vi "PPAS_Teleop_System_Execute.vi"(11 "Teleop Elapsed Seconds":dbl) -> ()   [LabVIEW 2019]
uses:
  <vilib>/Rock Robotics/WPI/Joystick/XBox Buttons Indexer.ctl
  <vilib>/Rock Robotics/WPI/Joystick/XBox Axes Indexer.ctl
  <vilib>/Rock Robotics/WPI/ThirdParty/JAS_Junk/TrajLib/TypeDef/CHASSIS_SPEEDS.ctl
  <vilib>/Rock Robotics/WPI/ThirdParty/JAS_Junk/TrajLib/VI/Util_GetTime_U32.vi
  <vilib>/Rock Robotics/WPI/ThirdParty/JAS_Junk/TrajLib/VI/numCmd_Send_Generic.vi
  <vilib>/Rock Robotics/WPI/ThirdParty/JAS_Junk/TrajLib/VI/BoolCmd_Send_Internal.vi
  <vilib>/Rock Robotics/WPI/ThirdParty/JAS_Junk/TrajLib/VI/numCmd_ObtainQueue_Generic.vi
  <vilib>/Rock Robotics/WPI/ThirdParty/JAS_Junk/TrajLib/VI/BoolCmd_ObtainQueue.vi
  <vilib>/Rock Robotics/WPI/ThirdParty/JAS_Junk/TrajLib/VI/Util_GetTime_U64.vi
  Swerve_Drive_System/PPAS_DRIVE_GLOBALS.vi
  <vilib>/Rock Robotics/WPI/Utilities/WPI_GetSetVariantRefNum.vi
  <vilib>/Rock Robotics/Network Tables/NT Write Integer Array.vi
  <vilib>/Rock Robotics/Network Tables/NT Write Numeric Array.vi
  <vilib>/Rock Robotics/Network Tables/NT Write Boolean Array.vi
  AutoCommand/PPAS_AUTOCMD_GLOBALS.vi
  <vilib>/Rock Robotics/WPI/ThirdParty/JAS_Junk/TrajLib/Trajectory_Library.lvlib
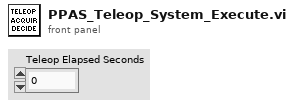
[diagram p1: front panel]
types:
  T1 = typedef "XBox Buttons Indexer.ctl" = enum16{"A", "B", "X", "Y", "Left Bumper", "Right Bumper", "Back", "Start", "Left Joystick", "Right Joystick"}
  T2 = typedef "XBox Axes Indexer.ctl" = enum16{"Left X", "Left Y", "Left Trigger", "Right Trigger", "Right X", "Right Y"}
  T3 = typedef "WPI_JoystickDevRef.ctl" = cluster{"Device":T4}
  T4 = typedef "WPI_JoystickDeviceEnum.ctl" = enum16{"USB 0", "USB 1", "USB 2", "USB 3", "USB 4", "USB 5"}
  T5 = typedef "Trajectory_Library.lvlib/CHASSIS_SPEEDS.ctl" = cluster{"vX":dbl, "vY":dbl, "vOmega":dbl}
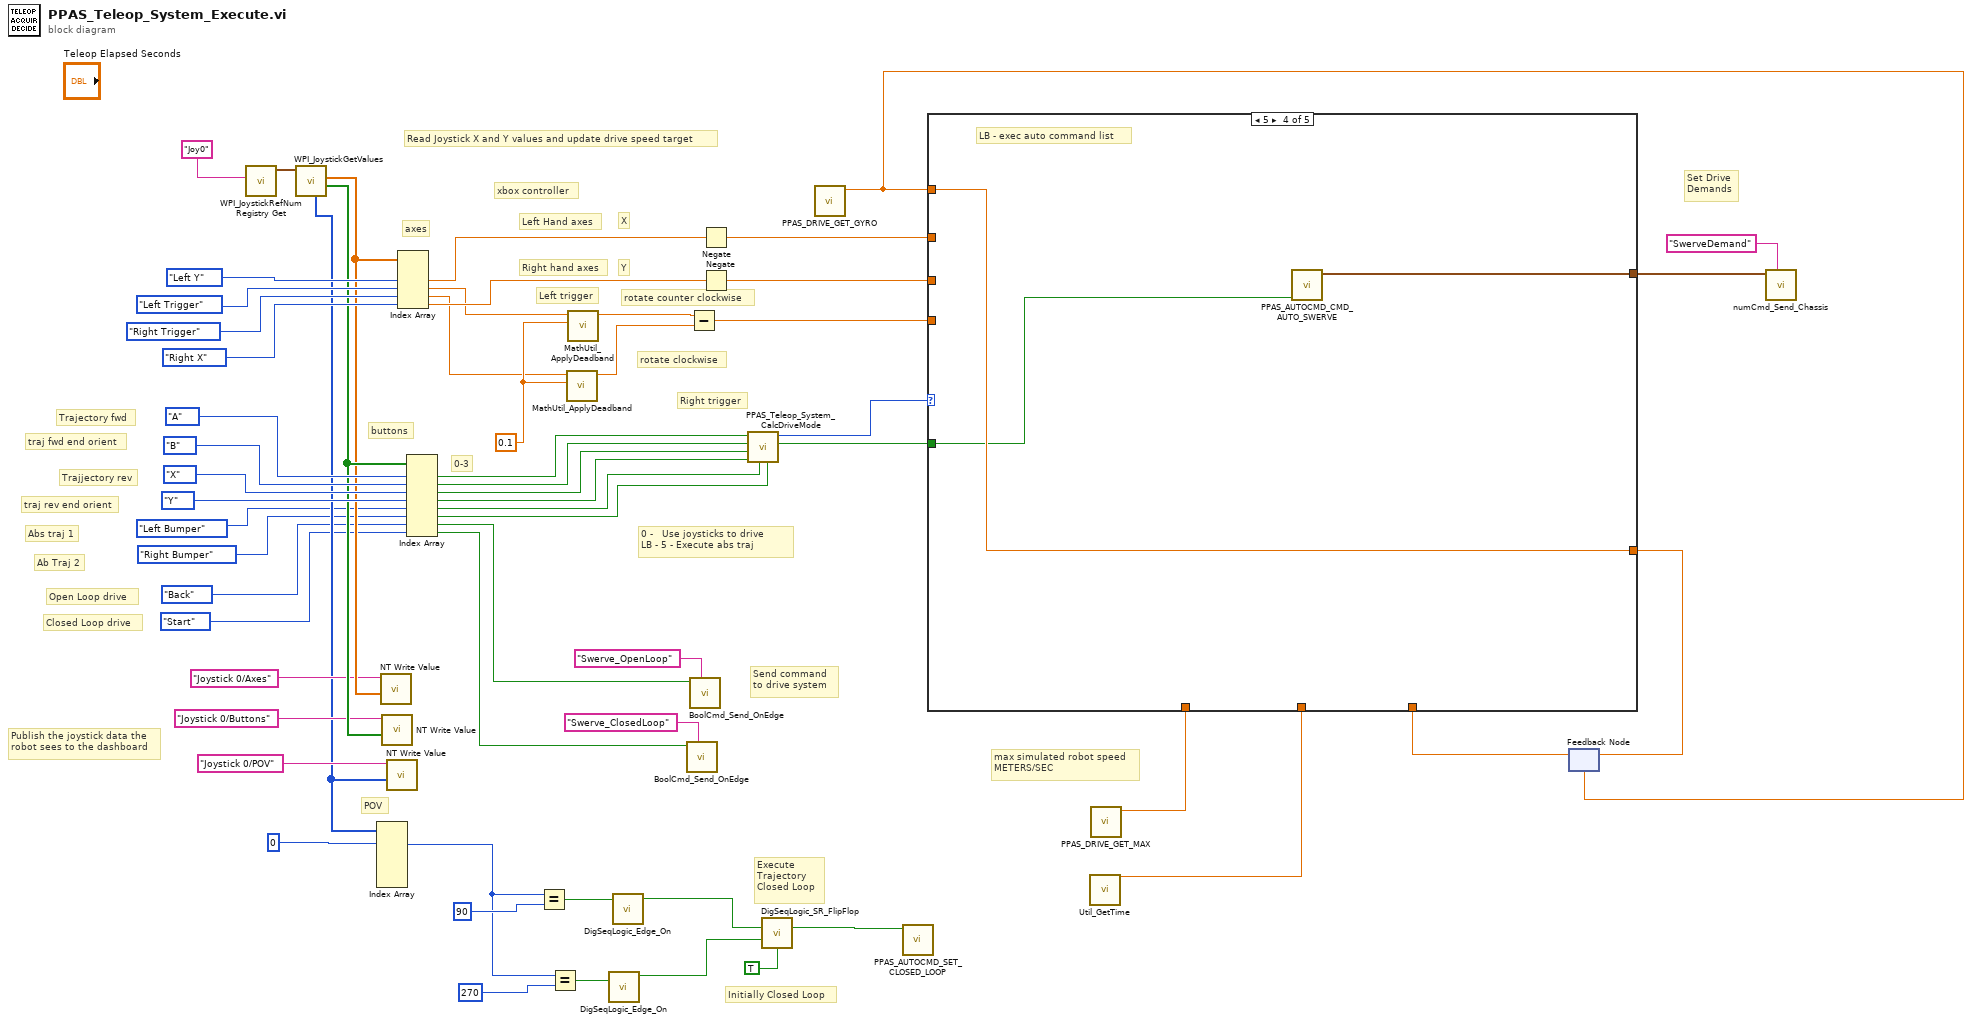
[diagram p0: block diagram]
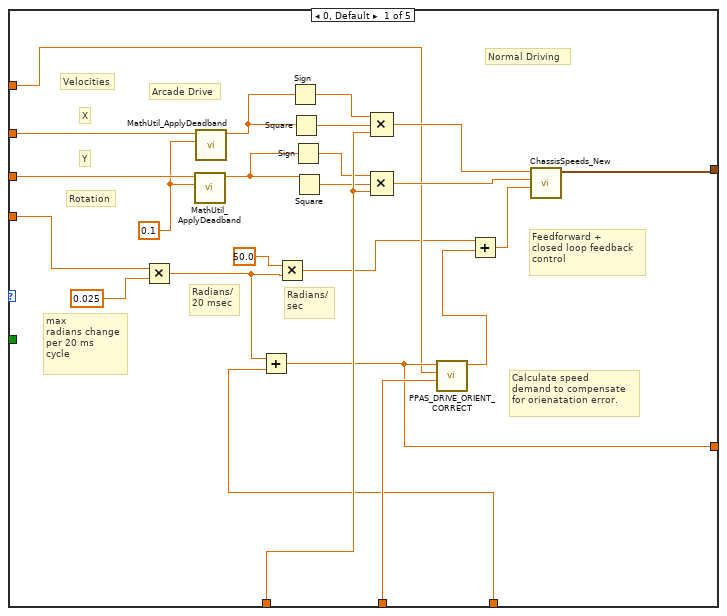
[diagram p2: hidden frame]
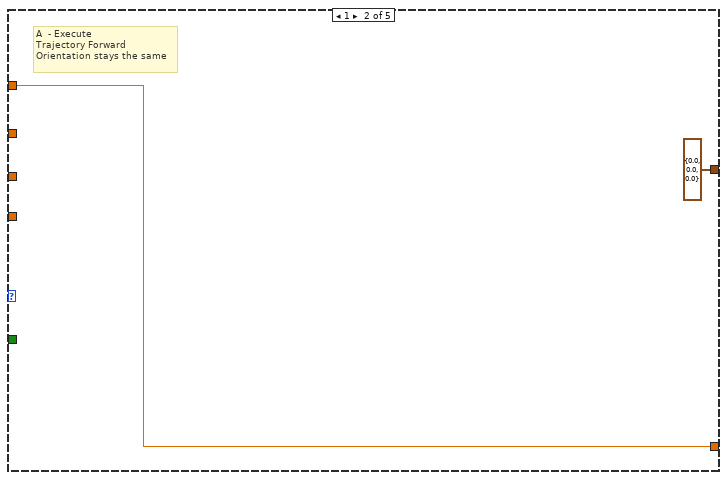
[diagram p3: hidden frame]
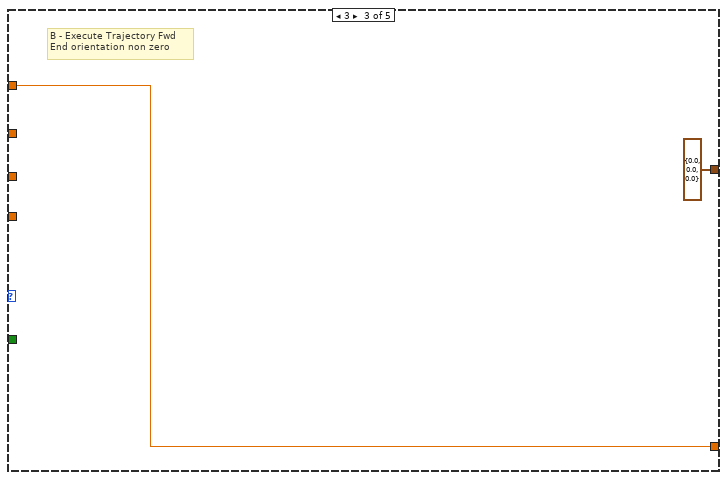
[diagram p4: hidden frame]
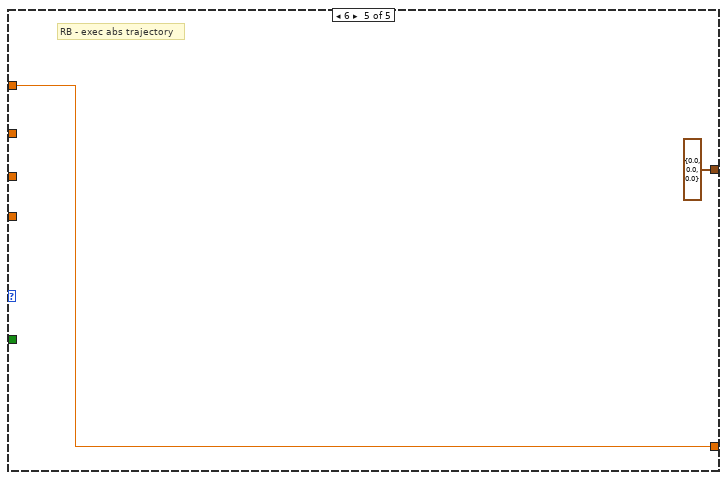
[diagram p5: hidden frame]
diagram:
  w48 = 0.1 ("Deadband")
  # "Send command\nto drive system"
  # "Ab Traj 2"
  # "Abs traj 1"
  # "POV"
  # "traj rev end orient"
  # "traj fwd end orient"
  # "Trajjectory rev"
  # "Closed Loop drive"
  # "Open Loop drive"
  # "Trajectory fwd"
  # "0 -   Use joysticks to drive\nLB - 5 - Execute abs traj"
  # "Execute\nTrajectory\nClosed Loop"
  # "Set Drive\nDemands"
  # "Initially Closed Loop"
  # "0-3"
  # "xbox controller"
  # "Left trigger"
  # "rotate counter clockwise"
  # "Right trigger"
  # "rotate clockwise"
  # "Left Hand axes"
  # "Right hand axes"
  # "Y"
  # "X"
  # "buttons"
  # "axes"
  # "max simulated robot speed\nMETERS/SEC"
  # "Publish the joystick data the\nrobot sees to the dashboard"
  # "Read Joystick X and Y values and update drive speed target"
  n1 = call <vilib>:"WPI_JoystickRefNum Registry Get.vi"("refnum name"="Joy0") -> ("JoystickDevRef"=w32:T3)  [unwired: 1 in, 9 out]
  n2 = call <vilib>:"WPI_JoystickGetValues.vi"("JoystickDevRef"=w32) -> ("Buttons"=w36:bool[], "Axes"=w35:dbl[], "POVs"=w19:i16[])  [unwired: 6 in, 2 out]
  n3 = Index Array(array=w19, index #1=0 ("index")) -> (element #1=w15:i16)  [unwired: 5 in, 5 out]
  n4 = call-poly <vilib>:"NT Write Value.vi"("value"=w35, "name"="Joystick 0/Axes" ("Name")) -> ()  [unwired: 9 in, 1 out]
  n5 = call-poly <vilib>:"NT Write Value.vi"("value"=w36, "name"="Joystick 0/Buttons" ("Name")) -> ()  [unwired: 9 in, 1 out]
  n6 = call-poly <vilib>:"NT Write Value.vi"("value"=w19, "name"="Joystick 0/POV" ("Name")) -> ()  [unwired: 9 in, 1 out]
  n7 = Index Array(array=w35, index #2=XBox_Axes_Indexer."Left Y" ("XBox Axes"), index #3=XBox_Axes_Indexer."Left Trigger" ("XBox Axes"), index #4=XBox_Axes_Indexer."Right Trigger" ("XBox Axes"), index #5=XBox_Axes_Indexer."Right X" ("XBox Axes")) -> (element #2=w44:dbl, element #3=w26:dbl, element #4=w24:dbl, element #5=w45:dbl)  [unwired: 1 in, 1 out]
  n8 = Index Array(array=w36, index #1=XBox_Buttons_Indexer."A" ("XBox Buttons"), index #2=XBox_Buttons_Indexer."B" ("XBox Buttons"), index #3=XBox_Buttons_Indexer."X" ("XBox Buttons"), index #4=XBox_Buttons_Indexer."Y" ("XBox Buttons"), index #5=XBox_Buttons_Indexer."Left Bumper" ("XBox Buttons"), index #6=XBox_Buttons_Indexer."Right Bumper" ("XBox Buttons"), index #7=XBox_Buttons_Indexer."Back" ("XBox Buttons"), index #8=XBox_Buttons_Indexer."Start" ("XBox Buttons")) -> (element #1=w37:bool, element #2=w46:bool, element #3=w47:bool, element #4=w55:bool, element #5=w6:bool, element #6=w5:bool, element #7=w2:bool, element #8=w1:bool)
  n9 = Equal?(x=w15, y=i16 90) -> (x = y?=w14:bool)
  n10 = Equal?(x=w15, y=i16 270) -> (x = y?=w13:bool)
  n11 = call <vilib>:"MathUtil_ApplyDeadband.vi"("Deadband"=w48, "Value"=w24) -> ("Result"=w23:dbl)  [unwired: 9 in]
  n12 = call <vilib>:"MathUtil_ApplyDeadband.vi"("Deadband"=w48, "Value"=w26) -> ("Result"=w25:dbl)  [unwired: 9 in]
  n13 = call <vilib>:"DigSeqLogic_Edge_On.vi"("Input"=w13) -> ("On Edge"=w11:bool)  [unwired: 10 in]
  n14 = call <vilib>:"DigSeqLogic_Edge_On.vi"("Input"=w14) -> ("On Edge"=w12:bool)  [unwired: 10 in]
  n15 = call <vilib>:"BoolCmd_Send_OnEdge.vi"("Command Name"="Swerve_ClosedLoop", "Value"=w1) -> ()  [unwired: 9 in, 1 out]
  n16 = Subtract(x=w25, y=w23) -> (x-y=w41:dbl)
  n17 = call <vilib>:"BoolCmd_Send_OnEdge.vi"("Command Name"="Swerve_OpenLoop", "Value"=w2) -> ()  [unwired: 9 in, 1 out]
  n18 = Negate(x=w44) -> (-x=w42:dbl)
  n19 = Negate(x=w45) -> (-x=w43:dbl)
  n20 = call "PPAS_Teleop_System_CalcDriveMode.vi"("Abs Traj 2"=w5, "Abs Traj 1"=w6, "Traj Rev Follow Orient"=w55, "Traj Rev Same Orient"=w47, "Traj Fwd Follow Orient"=w46, "Traj Fwd Same Orient"=w37) -> ("Dirve Mode Changed"=w39:bool, "Drive Mode"=w38:i32)  [unwired: 4 in]
  n21 = call <vilib>:"DigSeqLogic_SR_FlipFlop.vi"("Set"=w12, "Reset"=w11, "Initial Value"=TRUE) -> ("Output"=w50:bool)  [unwired: 11 in, 1 out]
  n22 = call "PPAS_DRIVE_GET_GYRO.vi"() -> ("Gyro Heading Radians"=w28:dbl)  [unwired: 11 in]
  n23 = call "PPAS_AUTOCMD_SET_CLOSED_LOOP.vi"("AUTO_CLOSED_LOOP"=w50) -> ()  [unwired: 11 in]
  n24 = call <vilib>:"Util_GetTime.vi"() -> ("FPGA_Time_Seconds"=w30:dbl)  [unwired: 9 in, 2 out]
  n25 = call "PPAS_DRIVE_GET_MAX.vi"() -> ("Max Wheel Vel (Meter/Sec)"=w40:dbl)  [unwired: 10 in, 1 out]
  n26 = feedback #1(w28) -> (w27:dbl)
  n27 = case shown="5" w38 {
    tunnel: w43 -> [w73 _ _ _ _]
    tunnel: w40 -> [w83 _ _ _ _]
    tunnel: w39 -> [_ _ _ w88 _]
    tunnel: w42 -> [w75 _ _ _ _]
    tunnel: w41 -> [w77 _ _ _ _]
    tunnel: w28 -> [w66 w85 w87 w90 w92]
    tunnel: [w69 T5 {"vX"=0.0, "vY"=0.0, "vOmega"=0.0} ("Chassis Velocity Target SI") T5 {"vX"=0.0, "vY"=0.0, "vOmega"=0.0} ("Chassis Velocity Target SI") w89 T5 {"vX"=0.0, "vY"=0.0, "vOmega"=0.0} ("Chassis Velocity Target SI")] -> w22
    tunnel: w30 -> [w68 _ _ _ _]
    tunnel: [w67 w85 w87 w90 w92] -> w29
    tunnel: w27 -> [w65 _ _ _ _]
    frame 0, Default {
      w72 = 0.1 ("Deadband")
      # "Feedforward +\nclosed loop feedback\ncontrol"
      # "Radians/\nsec"
      # "Radians/\n20 msec"
      # "Calculate speed\ndemand to compensate\nfor orienatation error."
      # "Normal Driving"
      # "Velocities"
      # "Rotation"
      # "max \nradians change\nper 20 ms\ncycle"
      # "Y"
      # "X"
      # "Arcade Drive"
      n28 = Multiply(x=w77, y=0.025) -> (x*y=w64:dbl)
      n29 = call <vilib>:"MathUtil_ApplyDeadband.vi"("Deadband"=w72, "Value"=w73) -> ("Result"=w76:dbl)  [unwired: 9 in]
      n30 = call <vilib>:"MathUtil_ApplyDeadband.vi"("Deadband"=w72, "Value"=w75) -> ("Result"=w74:dbl)  [unwired: 9 in]
      n31 = Add(x=w64, y=w65) -> (x+y=w67:dbl)
      n32 = Multiply(x=50.0, y=w64) -> (x*y=w61:dbl)
      n33 = Sign(1:w74) -> (0:w81:dbl)
      n34 = Square(x=w74) -> (x^2=w82:dbl)
      n35 = Sign(1:w76) -> (0:w79:dbl)
      n36 = Square(x=w76) -> (x^2=w80:dbl)
      n37 = Compound Arithmetic op=MULTIPLY(w81, w82, w83) -> (w71:dbl)
      n38 = Compound Arithmetic op=MULTIPLY(w79, w80, w83) -> (w70:dbl)
      n39 = call "PPAS_DRIVE_ORIENT_CORRECT.vi"("FPGA_Time_Seconds"=w68, "Gyro Heading Radians"=w66, "Drv Rotation Orentation Dmd  Radians"=w67) -> ("CO-ControlOutput"=w60:dbl)  [unwired: 8 in]
      n40 = Add(x=w61, y=w60) -> (x+y=w62:dbl)
      n41 = call <vilib>:"ChassisSpeeds_New.vi"("vAngular"=w62, "vY"=w70, "vX"=w71) -> ("CHASSIS"=w69:T5)  [unwired: 8 in]
    }
    frame 1 {
      # "A  - Execute\nTrajectory Forward\nOrientation stays the same"
    }
    frame 3 {
      # "B - Execute Trajectory Fwd \nEnd orientation non zero"
    }
    frame 5 {
      # "LB - exec auto command list"
      n42 = call "PPAS_AUTOCMD_CMD_AUTO_SWERVE.vi"("Init"=w88) -> ("Chassis Velocity Target SI"=w89:T5)  [unwired: 8 in, 2 out]
    }
    frame 6 {
      # "RB - exec abs trajectory"
    }
  }
  n43 = feedback-in #1(w29) -> ()
  n44 = call <vilib>:"numCmd_Send_Chassis.vi"("Command Name"="SwerveDemand", "Chassis Speeds"=w22) -> ()  [unwired: 9 in, 1 out]
